vi "Read Controlled Devices.vi"(0 "Arduino in":refnum<class "Arduino.lvclass">, 11 "error in (no error)":errorcluster) -> (4 "Arduino out":refnum<class "Arduino.lvclass">, 6 "Controlled Devices":T1(array[cluster]), 8 "Device Cols":cluster{"col_index":dbl, "param_count":dbl}[](array[cluster]), 15 "error out":errorcluster)   [LabVIEW 2013, in "Arduino.lvclass"]
uses:
  Arduino.lvclass
  Arduino.lvclass/Arduino.ctl
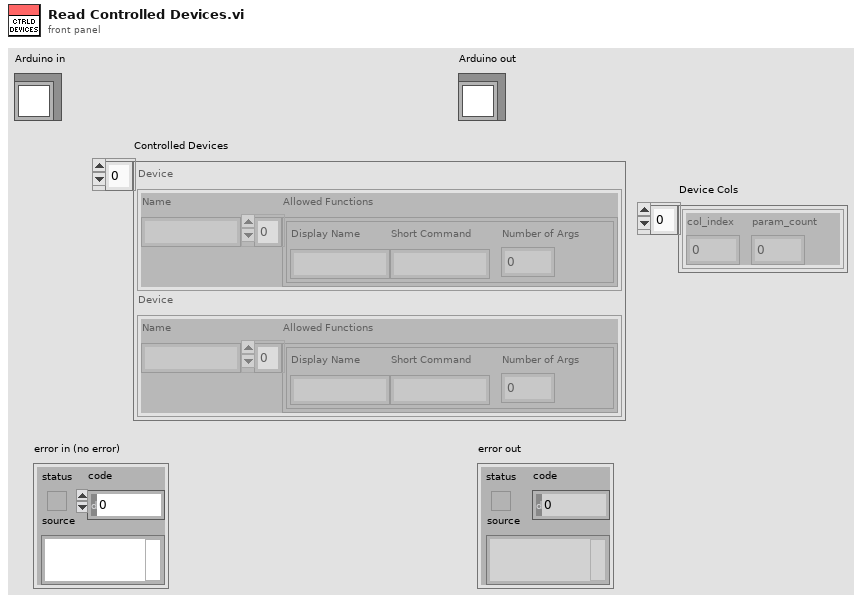
[diagram p1: front panel]
types:
  T1 = cluster{"Name":string, "Allowed Functions":cluster{"Display Name":string, "Short Command":string, "Number of Args":dbl}[]}[]
  T2 = cluster{"Display Name":string, "Short Command":string, "Number of Args":dbl}[]
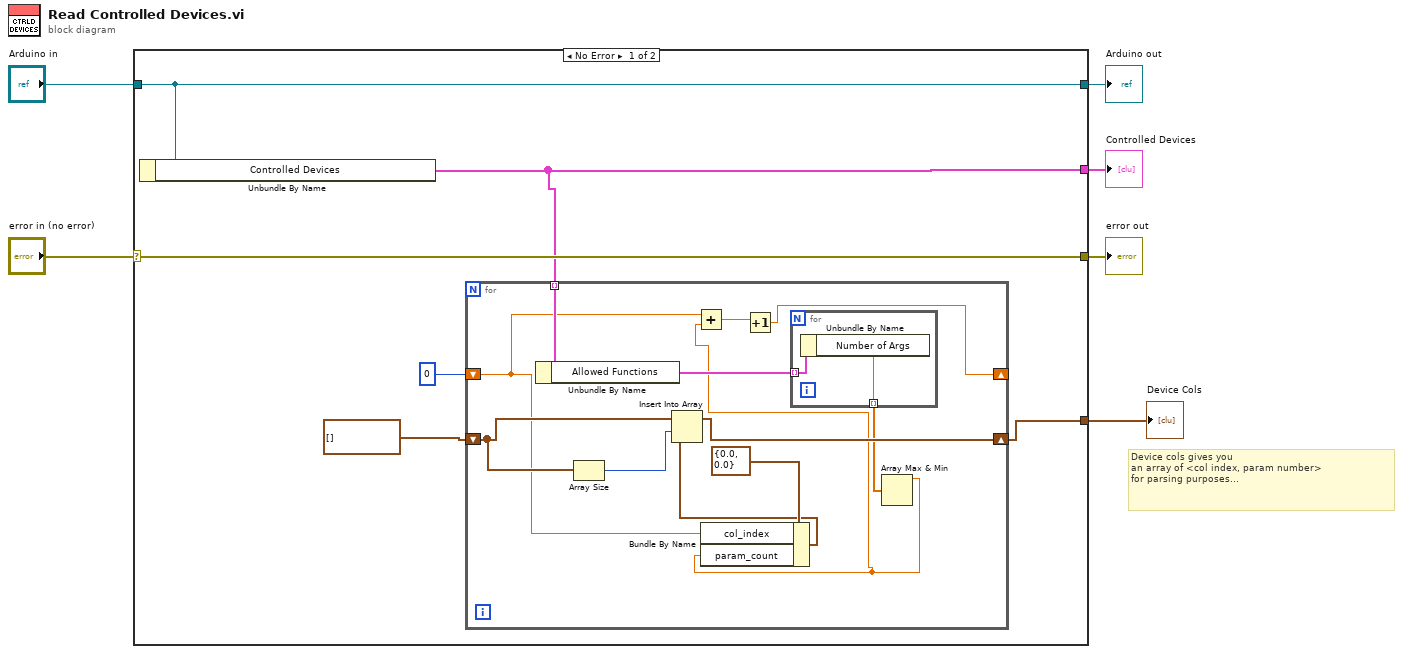
[diagram p0: block diagram]
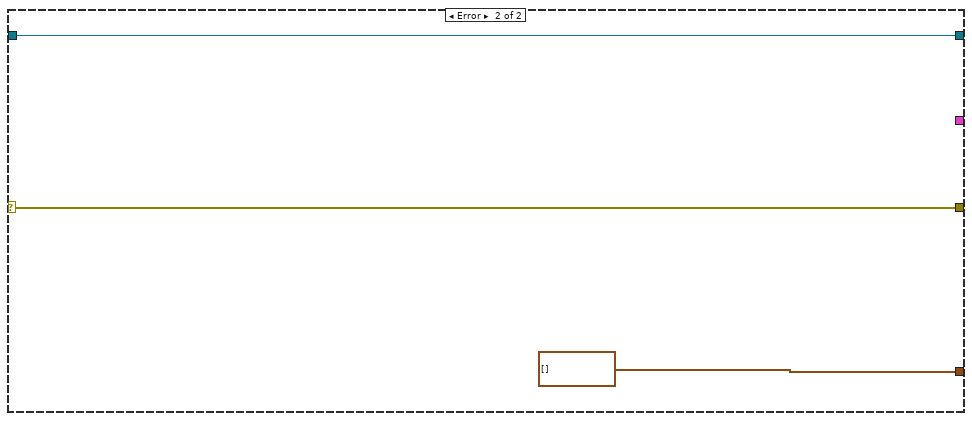
[diagram p2: hidden frame]
diagram:
  # "Device cols gives you\nan array of <col index, param number>\nfor parsing purposes..."
  n1 = case shown="No Error" "error in (no error)" {
    selector: "error in (no error)" -> [w12 w28]
    tunnel: [w12 w28] -> w5
    tunnel: [w11 w29] -> w3
    tunnel: "Arduino in" -> [w11 w29]
    tunnel: [w10 _] -> w2
    tunnel: [w8 cluster{"col_index":dbl, "param_count":dbl}[] [] ("Device Cols")] -> w1
    frame No Error {
      n2 = Unbundle By Name(w11) -> ("Controlled Devices"=w10:T1)
      n3 = for {
        tunnel: w10 -> [w21] mode=indexing
        shift-right: [w22] -> w8
        shift-left: cluster{"col_index":dbl, "param_count":dbl}[] [] ("Device Cols") -> [w23]
        shift-right: [w13] -> _
        shift-left: 0 -> [w16]
        n4 = Unbundle By Name(w21) -> ("Allowed Functions"=w20:T2)
        n5 = Array Size(array=w23) -> (size(s)=w24:i32)
        n6 = for {
          tunnel: w20 -> [w26] mode=indexing
          tunnel: [w25] -> w19 mode=indexing
          n7 = Unbundle By Name(w26) -> ("Number of Args"=w25:dbl)
        }
        n8 = Array Max & Min(array=w19) -> (max value=w15:dbl)  [unwired: 3 out]
        n9 = Add(x=w16, y=w15) -> (x+y=w14:dbl)
        n10 = Bundle By Name(cluster=cluster{"col_index":dbl, "param_count":dbl} {"col_index"=0.0, "param_count"=0.0} ("Cluster"), "col_index"=w16, "param_count"=w15) -> (w17:cluster{"col_index":dbl, "param_count":dbl})
        n11 = Insert Into Array(array=w23, index=w24, new element=w17) -> (w22:cluster{"col_index":dbl, "param_count":dbl}[])
        n12 = Increment(x=w14) -> (x+1=w13:dbl)
      }
    }
    frame Error {
    }
  }
  "error out" <- w5
  "Arduino out" <- w3
  "Controlled Devices" <- w2
  "Device Cols" <- w1
